vi "Get Member Data from Private Data Control.vi"(7 "AppInst":refnum<vi>, 8 "error in (no error)":errorcluster, 10 "Target Path":path) -> (0 "error out":errorcluster, 1 "Controls":refnum<vi>[](array[refnum]), 2 "Private data Control":refnum<vi>)   [LabVIEW 2020, in "Message Maker.lvlib"]
uses:
  Message Maker.lvlib
  <vilib>/Utility/traverseref.llb/TRef TravTarget.ctl
  <vilib>/Utility/traverseref.llb/VI Scripting - Traverse.lvlib
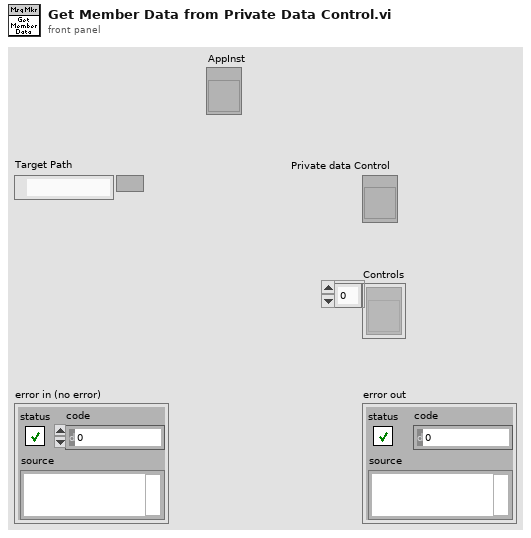
[diagram p1: front panel]
types:
  T1 = typedef "TRef TravTarget.ctl" = enum16{"FP", "BD", "Other"}
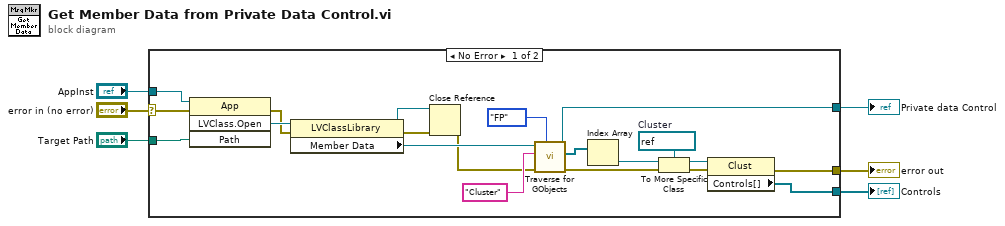
[diagram p0: block diagram]
diagram:
  n1 = case shown="No Error" "error in (no error)" {
    selector: "error in (no error)" -> [w23 w27]
    tunnel: [w11 w27] -> w6
    tunnel: "Target Path" -> [w24 _]
    tunnel: "AppInst" -> [w22 _]
    tunnel: [w7 _] -> w2
    tunnel: [w9 _] -> w1
    frame No Error {
      w15 = refnum<vi> refnum  # Cluster
      n2 = invoke class="App" method="LVClass.Open"(reference=w22, error in=w23, "Path"=w24) -> (error out=w25:errorcluster, "LVClass.Open"=w26:refnum<vi>)  [unwired: 1 in, 2 out]
      n3 = property class="LVClassLibrary"(reference=w26, error in=w25) -> (reference out=w10:refnum<vi>, error out=w21:errorcluster, "Member Data"=w20:refnum<vi>)
      n4 = Close Reference(reference=w10, error in (no error)=w21) -> (error out=w8:errorcluster)
      n5 = call <vilib>:"Traverse for GObjects.vi"("Traverse Target"=TRef_TravTarget."FP", "error in (no error)"=w8, "Class Name"="Cluster", "VI Refnum"=w20) -> ("error out"=w12:errorcluster, "References"=w17:refnum<vi>[], "dup VI Refnum"=w9:refnum<vi>)  [unwired: 4 in, 1 out]
      n6 = Index Array(array=w17) -> (element=w16:refnum<vi>)  [unwired: 1 in]
      n7 = To More Specific Class(target class=w15, reference=w16, error in=w12) -> (specific class reference=w14:refnum<vi>, error out=w13:errorcluster)
      n8 = property class="Clust"(reference=w14, error in=w13) -> (error out=w11:errorcluster, "Controls[]"=w7:refnum<vi>[])  [unwired: 1 out]
    }
    frame Error {
    }
  }
  "error out" <- w6
  "Controls" <- w2
  "Private data Control" <- w1
